vi "Find Local NHMFL ENET Address.vi"(8 "error in (no error)":errorcluster, 10 "Search Reg Exp (NHMFL)":string="^146\\.201\\.") -> (0 "error out":errorcluster, 2 "Address Dot Notation":string, 3 "Ethernet Address":u32 format="%.0x")   [LabVIEW 2025]
doc: "Author: Scott Hannahs <sth@magnet.fsu.edu>\n\nAuthor: Scott Hannahs <sth@magnet.fsu.edu>\n\nThis software is licensed for use under the “MIT License\"\nCopyright (c) 2025 Scott Hannahs, sth@sth@magnet.sthnet.net\n\nPermission is hereby granted, free of charge, to any person obtaining a copy of this software and associated documentation files (the \"Software\"), to deal in the Software without restriction, including without limitation the rights to use, copy, modify, merge, publish, distribute, sublicense, and/or sell copies of the Software, and to permit persons to whom the Software is furnished to do so, subject to the following conditions: The above copyright notice and this permission notice shall be included in all copies or substantial portions of the Software.\n\nTHE SOFTWARE IS PROVIDED \"AS IS\", WITHOUT WARRANTY OF ANY KIND, EXPRESS OR IMPLIED, INCLUDING BUT NOT LIMITED TO THE WARRANTIES OF MERCHANTABILITY, FITNESS FOR A PARTICULAR PURPOSE AND NONINFRINGEMENT. IN NO EVENT SHALL THE AUTHORS OR COPYRIGHT HOLDERS BE LIABLE FOR ANY CLAIM, DAMAGES OR OTHER LIABILITY, WHETHER IN AN ACTION OF CONTRACT, TORT OR OTHERWISE, ARISING FROM, OUT OF OR IN CONNECTION WITH THE SOFTWARE OR THE USE OR OTHER DEALINGS IN THE SOFTWARE."
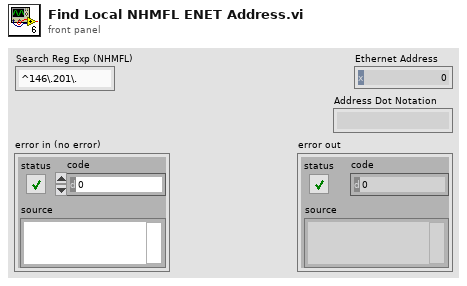
[diagram p1: front panel]
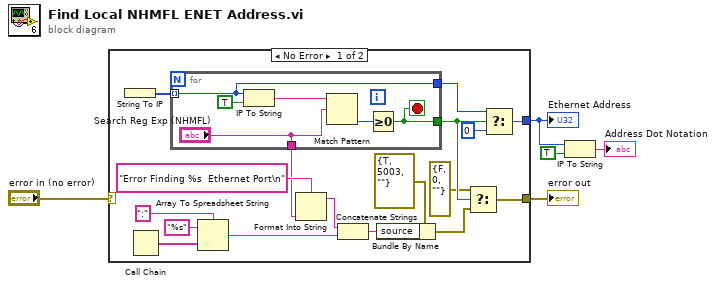
[diagram p0: block diagram]
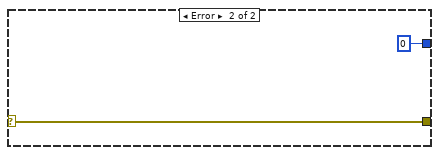
[diagram p2: hidden frame]
diagram:
  n1 = case shown="No Error" "error in (no error)" {
    selector: "error in (no error)" -> [_ w29]
    tunnel: [w21 u32 0 ("f")] -> w2
    tunnel: [w17 w29] -> w4
    frame No Error {
      n2 = String To IP() -> (0:w22:u32[])  [unwired: 1 in]
      n3 = Call Chain() -> (call chain=w10:string[])
      n4 = for {
        tunnel: w22 -> [w28] mode=indexing
        tunnel: [w28] -> w20
        tunnel: [w24] -> w18
        tunnel: ["Search Reg Exp (NHMFL)"] -> w11
        stop <- w24 stop-if-true
        n5 = IP To String(1:TRUE ("dot notation? (F)"), 2:w28) -> (0:w26:string)
        n6 = Match Pattern(string=w26, regular expression="Search Reg Exp (NHMFL)") -> (offset past match=w25:i32)  [unwired: 1 in, 3 out]
        n7 = Greater Or Equal To 0?(x=w25) -> (x >= 0?=w24:bool)
      }
      n8 = Array To Spreadsheet String(delimiter (Tab)=":", array=w10, 3:"%s" ("format string")) -> (spreadsheet string=w6:string)
      n9 = Format Into String(format string="Error Finding %s  Ethernet Port\n" ("source"), w11) -> (resulting string=w15:string)  [unwired: 2 in, 1 out]
      n10 = Concatenate Strings(w15, w6) -> (w7:string)
      n11 = Bundle By Name(cluster=errorcluster {"status"=TRUE, "code"=5003, "source"=""} ("f"), "source"=w7) -> (w13:errorcluster)
      n12 = Select(t=errorcluster {"status"=FALSE, "code"=0, "source"=""} ("error IO"), s=w18, f=w13) -> (s? t:f=w17:errorcluster)
      n13 = Select(t=w20, s=w18, f=u32 0) -> (s? t:f=w21:u32)
    }
    frame Error {
    }
  }
  "Ethernet Address" <- w2
  "error out" <- w4
  n14 = IP To String(1:TRUE ("dot notation? (F)"), 2:w2) -> (0:→"Address Dot Notation":string)
